vi "test Process Records with Timestamps.vi"(8 "error in":errorcluster, 11 "TestCase in":refnum<class "Engine.lvclass">) -> (0 "error out":errorcluster, 3 "TestCase out":refnum<class "Engine.lvclass">)   [LabVIEW 2020, in "Engine.lvclass"]
uses:
  Engine.lvclass
  Shared/RT Hardware Channel Settings.ctl
  Shared/RT Label Settings.ctl
  Shared/Label.ctl
  Shared/RT Parameters.ctl
  Shared/Parameter Definition.ctl
  <vilib>/NI/NI VeriStand Encoding and Decoding/Encoding.ctl
  <vilib>/NI VeriStand/Custom Device API/Custom Device Item Ref.ctl
  Shared/Transfer Type.ctl
  <vilib>/NI VeriStand/Custom Device API/Data Reference.ctl
  <instrlib>/BTICardLib/Public/Controls/429 Record.ctl
  Shared/Map of Identifiers to Indexes.ctl
  <vilib>/addons/_JKI Toolkits/VI Tester/TestCase.llb/TestCase.lvclass
  <instrlib>/BTICardLib/BTICardLV.lvlib
  <vilib>/NI VeriStand/Custom Device API/Custom Device API.lvlib
  <vilib>/NI/NI VeriStand Encoding and Decoding/Encoding and Decoding.lvlib
  Engine/Custom Device/Custom Device.lvlib
  C:/Program Files (x86)/National Instruments/LabVIEW 2020/vi.lib/addons/_JKI Toolkits/VI Tester/TestCase.llb/TestCase.lvclass
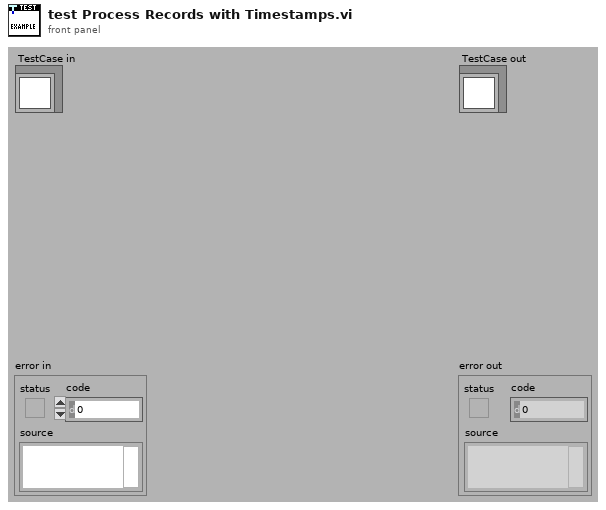
[diagram p1: front panel]
types:
  T1 = typedef "BTICardLV.lvlib/429 Record.ctl" = cluster{"type":u16, "count":u16, "timestamp":u32, "msgact":u16, "decgap":u16, "data":u32, "timestamph":u32}
  T2 = typedef "RT Hardware Channel Settings.ctl" = cluster{"channel #":u16, "channel handle":u64, "labels settings for RT":T3[]}
  T3 = typedef "RT Label Settings.ctl" = cluster{"Name":string, "xmlName":string, "label":T4, "transfer period":u32, "SDI_Enabled":bool, "SDI":u8, "parameter driver data":T5, "transfer type":T9, "has timestamp?":bool, "Label Disable/Trigger Channel Reference":T8, "Message Handle":u64, "Initialized?":bool, "Word Initial Raw Value":u32, "Label Timestamp Channel Data Reference":T10, "disabled":bool}
  T4 = typedef "Label.ctl" = u8
  T5 = typedef "RT Parameters.ctl" = cluster{"parameter definitions":T6[], "Tx parameter refs":T8[]}
  T6 = typedef "Parameter Definition.ctl" = cluster{"start index":i32, "size":i32, "encoding":T7, "signed":bool, "scale multiplier":dbl, "scale offset":dbl}
  T7 = typedef "Encoding and Decoding.lvlib/Encoding.ctl" = enum16{"BNR", "BCD", "Discrete"}
  T8 = typedef "Custom Device API.lvlib/Custom Device Item Ref.ctl" = u64
  T9 = typedef "Transfer Type.ctl" = enum16{"Scheduled", "Acyclic", "Block", "Strobe"}
  T10 = typedef "Custom Device API.lvlib/Data Reference.ctl" = i32
  T11 = typedef "Map of Identifiers to Indexes.ctl" = map{cluster{"Port":u8, "Label":u8, "SDI":u8}, cluster{"channel index":i32, "label index":i32, "start index":i32, "parameters":i32, "timestamp index":i32}}
  T12 = map{cluster{"hardware channel":u8, "label":u8, "SDI":u8}, cluster{"data word":u32, "time stamp":dbl}}
  T13 = cluster{"hardware channel":u8, "label":u8, "SDI":u8}
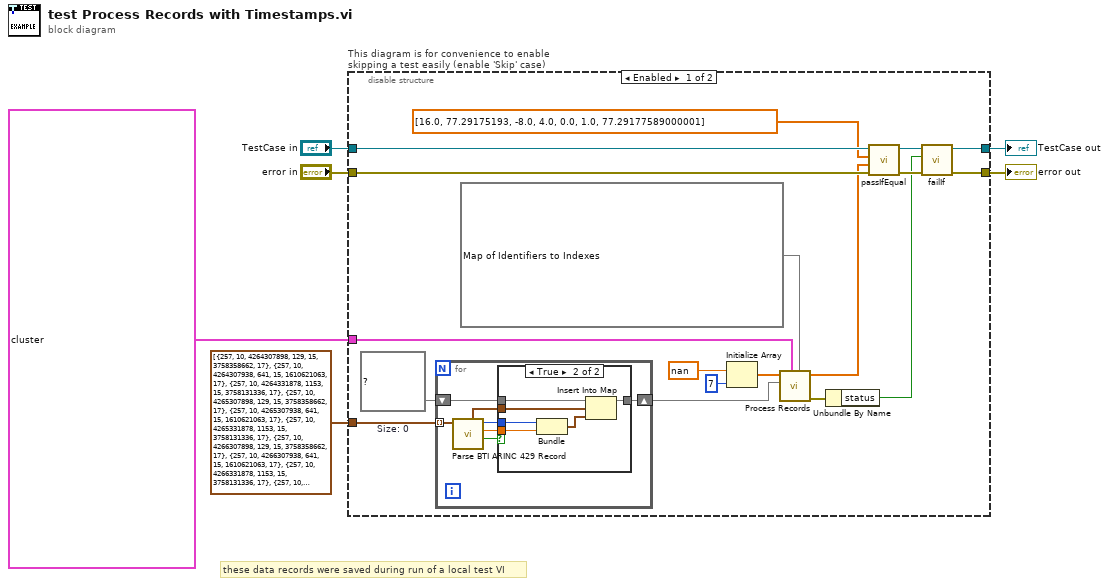
[diagram p0: block diagram]
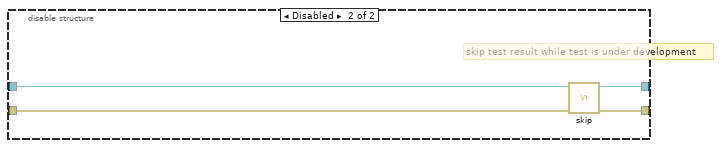
[diagram p3: hidden frame]
diagram:
  # "these data records were saved during run of a local test VI"
  n1 = disable-structure "This diagram is for convenience to enable skipping a test easily (enable 'Skip' case)" shown="Enabled" {
    disable-tunnel: "TestCase in" -> [w20 w42]
    disable-tunnel: [w24 w40] -> w3
    disable-tunnel: [w23 w41] -> w5
    disable-tunnel: "error in" -> [w19 w39]
    disable-tunnel: T2[] data[160728B] ("RT hardware channel data") -> [w11 _]
    disable-tunnel: T1[] [{"type"=257, "count"=10, "timestamp"=4264307898, "msgact"=129, "decgap"=15, "data"=3758358662, "timestamph"=17}, {"type"=257, "count"=10, "timestamp"=4264307938, "msgact"=641, "decgap"=15, "data"=1610621063, "timestamph"=17}, {"type"=257, "count"=10, "timestamp"=4264331878, "msgact"=1153, "decgap"=15, "data"=3758131336, "timestamph"=17}, {"type"=257, "count"=10, "timestamp"=4265307898, "msgact"=129, "decgap"=15, "data"=3758358662, "timestamph"=17}, {"type"=257, "count"=10, "timestamp"=4265307938, "msgact"=641, "decgap"=15, "data"=1610621063, "timestamph"=17}, {"type"=257, "count"=10, "timestamp"=4265331878, "msgact"=1153, "decgap"=15, "data"=3758131336, "timestamph"=17}, {"type"=257, "count"=10, "timestamp"=4266307898, "msgact"=129, "decgap"=15, "data"=3758358662, "timestamph"=17}, {"type"=257, "count"=10, "timestamp"=4266307938, "msgact"=641, "decgap"=15, "data"=1610621063, "timestamph"=17}, {"type"=257, "count"=10, "timestamp"=4266331878, "msgact"=1153, "decgap"=15, "data"=3758131336, "timestamph"=17}, {"type"=257, "count"=10, "timestamp"=4267307898, "msgact"=129, "decgap"=15, "data"=3758358662, "timestamph"=17}, {"type"=257, "count"=10, "timestamp"=4267307938, "msgact"=641, "decgap"=15, "data"=1610621063, "timestamph"=17}, {"type"=257, "count"=10, "timestamp"=4267331858, "msgact"=1153, "decgap"=15, "data"=3758131336, "timestamph"=17}, {"type"=257, "count"=10, "timestamp"=4268307898, "msgact"=129, "decgap"=15, "data"=3758358662, "timestamph"=17}, {"type"=257, "count"=10, "timestamp"=4268307938, "msgact"=641, "decgap"=15, "data"=1610621063, "timestamph"=17}, {"type"=257, "count"=10, "timestamp"=4268331858, "msgact"=1153, "decgap"=15, "data"=3758131336, "timestamph"=17}, {"type"=257, "count"=10, "timestamp"=4269307898, "msgact"=129, "decgap"=15, "data"=3758358662, "timestamph"=17}, {"type"=257, "count"=10, "timestamp"=4269307938, "msgact"=641, "decgap"=15, "data"=1610621063, "timestamph"=17}, {"type"=257, "count"=10, "timestamp"=4269331858, "msgact"=1153, "decgap"=15, "data"=3758131336, "timestamph"=17}, {"type"=257, "count"=10, "timestamp"=4270307898, "msgact"=129, "decgap"=15, "data"=3758358662, "timestamph"=17}, {"type"=257, "count"=10, "timestamp"=4270307938, "msgact"=641, "decgap"=15, "data"=1610621063, "timestamph"=17}, {"type"=257, "count"=10, "timestamp"=4270331878, "msgact"=1153, "decgap"=15, "data"=3758131336, "timestamph"=17}, {"type"=257, "count"=10, "timestamp"=4271307898, "msgact"=129, "decgap"=15, "data"=3758358662, "timestamph"=17}, {"type"=257, "count"=10, "timestamp"=4271307938, "msgact"=641, "decgap"=15, "data"=1610621063, "timestamph"=17}, {"type"=257, "count"=10, "timestamp"=4271331858, "msgact"=1153, "decgap"=15, "data"=3758131336, "timestamph"=17}, {"type"=257, "count"=10, "timestamp"=4272307898, "msgact"=129, "decgap"=15, "data"=3758358662, "timestamph"=17}, {"type"=257, "count"=10, "timestamp"=4272307938, "msgact"=641, "decgap"=15, "data"=1610621063, "timestamph"=17}, {"type"=257, "count"=10, "timestamp"=4272331858, "msgact"=1153, "decgap"=15, "data"=3758131336, "timestamph"=17}, {"type"=257, "count"=10, "timestamp"=4273307898, "msgact"=129, "decgap"=15, "data"=3758358662, "timestamph"=17}, {"type"=257, "count"=10, "timestamp"=4273307938, "msgact"=641, "decgap"=15, "data"=1610621063, "timestamph"=17}, {"type"=257, "count"=10, "timestamp"=4273331878, "msgact"=1153, "decgap"=15, "data"=3758131336, "timestamph"=17}, {"type"=257, "count"=10, "timestamp"=4274307898, "msgact"=129, "decgap"=15, "data"=3758358662, "timestamph"=17}, {"type"=257, "count"=10, "timestamp"=4274307938, "msgact"=641, "decgap"=15, "data"=1610621063, "timestamph"=17}, {"type"=257, "count"=10, "timestamp"=4274331858, "msgact"=1153, "decgap"=15, "data"=3758131336, "timestamph"=17}, {"type"=257, "count"=10, "timestamp"=4275307898, "msgact"=129, "decgap"=15, "data"=3758358662, "timestamph"=17}, {"type"=257, "count"=10, "timestamp"=4275307938, "msgact"=641, "decgap"=15, "data"=1610621063, "timestamph"=17}, {"type"=257, "count"=10, "timestamp"=4275331858, "msgact"=1153, "decgap"=15, "data"=3758131336, "timestamph"=17}, {"type"=257, "count"=10, "timestamp"=4276307898, "msgact"=129, "decgap"=15, "data"=3758358662, "timestamph"=17}, {"type"=257, "count"=10, "timestamp"=4276307938, "msgact"=641, "decgap"=15, "data"=1610621063, "timestamph"=17}, {"type"=257, "count"=10, "timestamp"=4276331858, "msgact"=1153, "decgap"=15, "data"=3758131336, "timestamph"=17}, {"type"=257, "count"=10, "timestamp"=4277307898, "msgact"=129, "decgap"=15, "data"=3758358662, "timestamph"=17}, {"type"=257, "count"=10, "timestamp"=4277307938, "msgact"=641, "decgap"=15, "data"=1610621063, "timestamph"=17}, {"type"=257, "count"=10, "timestamp"=4277331858, "msgact"=1153, "decgap"=15, "data"=3758131336, "timestamph"=17}] ("records") -> [w10 _]
    frame Enabled {
      w9 = T12 {}  # Size: 0
      n2 = for {
        tunnel: w10 -> [w31] mode=indexing
        shift-right: [w28] -> w8
        shift-left: w9 -> [w29]
        n3 = call "Parse BTI ARINC 429 Record.vi"("record"=w31) -> ("hit"=w25:bool, "time stamp"=w30:dbl, "data word"=w26:u32, "message info"=w27:T13)  [unwired: 5 in, 2 out]
        n4 = case shown="True" w25 {
          tunnel: w29 -> [w32 w37]
          tunnel: [w32 w38] -> w28
          tunnel: w27 -> [_ w36]
          tunnel: w26 -> [_ w35]
          tunnel: w30 -> [_ w33]
          frame False {
          }
          frame True {
            n5 = Bundle("data word"=w35, "time stamp"=w33) -> (w34:cluster{"data word":u32, "time stamp":dbl})  [unwired: 1 in]
            n6 = Insert Into Map(map in=w37, key=w36, value=w34) -> (map out=w38:T12)  [unwired: 2 out]
          }
        }
      }
      n7 = Initialize Array(nan ("element"), 7 ("dimension size")) -> (w14:dbl[])
      n8 = call "Process Records.vi"("map from message info to indexes"=T11 {{"Port"=0, "Label"=134, "SDI"=0}={"channel index"=0, "label index"=134, "start index"=0, "parameters"=1, "timestamp index"=1}, {"Port"=2, "Label"=135, "SDI"=0}={"channel index"=2, "label index"=135, "start index"=2, "parameters"=1, "timestamp index"=-1}, {"Port"=4, "Label"=136, "SDI"=0}={"channel index"=4, "label index"=136, "start index"=3, "parameters"=3, "timestamp index"=6}} ("map"), "RT hardware channel data"=w11, "map from message info to data word"=w8, "parameter values in"=w14) -> ("error out"=w18:errorcluster, "parameter values out"=w13:dbl[])  [unwired: 4 in]
      n9 = Unbundle By Name(w18) -> ("status"=w17:bool)
      n10 = call-dynamic "passIfEqual.vi"("error in (no error)"=w19, "y"=w13, "x"=dbl[] [16.0, 77.29175193, -8.0, 4.0, 0.0, 1.0, 77.29177589000001] ("parameter values out"), "TestCase in"=w20) -> ("error out"=w21:errorcluster, "TestCase out"=w22:refnum<class "Engine.lvclass">)  [unwired: 6 in]
      n11 = call-dynamic "failIf.vi"("error in (no error)"=w21, "fail"=w17, "TestCase in"=w22) -> ("error out"=w23:errorcluster, "TestCase out"=w24:refnum<class "Engine.lvclass">)  [unwired: 7 in]
    }
    frame Disabled {
      # "skip test result while test is under development"
      n12 = call <vilib>:"skip.vi"("error in (no error)"=w39, "TestCase in"=w42) -> ("error out"=w41:errorcluster, "TestCase out"=w40:refnum<class "Engine.lvclass">)  [unwired: 8 in]
    }
  }
  "error out" <- w5
  "TestCase out" <- w3
